vi "Nodo_propiedad_implicito.vi"() -> ()   [LabVIEW 2016]
panel:
  in  "Array 2":string[](array[string])
  in  "Menu Ring 2":u16(ring) items=["PABLO", "LEOPOLDO", "ANDRES", "SANDRA"]
  in  "Menu Ring":u16(ring) items=["ERICK", "JUAN", "RENE", "JACOBO"]
  in  "Array":string[](array[string])
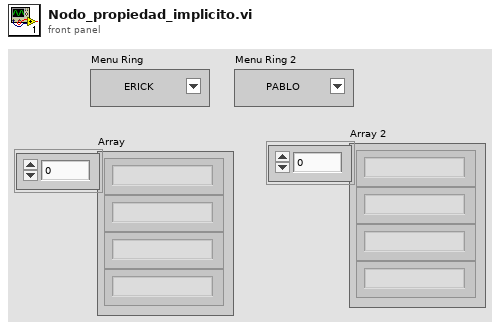
[diagram p1: front panel]
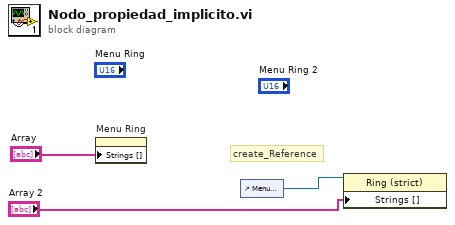
[diagram p0: block diagram]
diagram:
  # "create_Reference"
  n1 = property on="Menu Ring" class="Ring (strict)"("Strings []"="Array") -> ()  [unwired: 2 in, 2 out]
  n2 = control-ref of="Menu Ring 2"() -> (w2:refnum<vi>)
  n3 = property on="Property Node" class="Ring (strict)"(reference=w2, "Strings []"="Array 2") -> ()  [unwired: 1 in, 2 out]
